vi "RefreshXYGraphV2.vi"(8 "error in (no error)":errorcluster caption="entrée d'erreur (pas d'erreur)", 9 "Graph Index":i32, 11 "Interface en entrée":refnum<class "Interface.lvclass"> caption="DNL_LabVIEW Object in") -> (0 "error out":errorcluster caption="sortie d'erreur", 1 "CurvesInd":i32[](array[numeric]), 2 "XYGraph_Ref":refnum<vi>, 3 "Interface en sortie":refnum<class "Interface.lvclass"> caption="DNL_LabVIEW Object out")   [LabVIEW 2010, in "Interface.lvclass"]
uses:
  Interface.lvclass
  Interface.lvclass/Interface.ctl
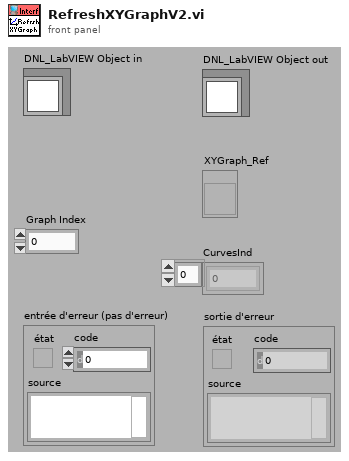
[diagram p1: front panel]
types:
  T1 = typedef "Interface.lvclass/CurveSetup.ctl" = cluster{"CurveName":string, "YParam":string, "XParam":string, "ZParam ":string, "GroupName":string, "LinWdth":u8, "PntCol":u32, "LinCol":u32, "LablFor":u8, "XScale":u32, "YScale":u32, "Interpol":u8, "DisplayName":string, "FillType":i16, "LineStyle":u8, "PntStyle":u8, "BarTyp":u8, "GraphIndex":i32, "Visible":bool, "XScaleName":string, "YScaleName":string, "XYGraph_Ref":refnum<vi>, "Data Only":bool, "DataQ Ref":refnum<queue>, "XParQ Ref":refnum<queue>}
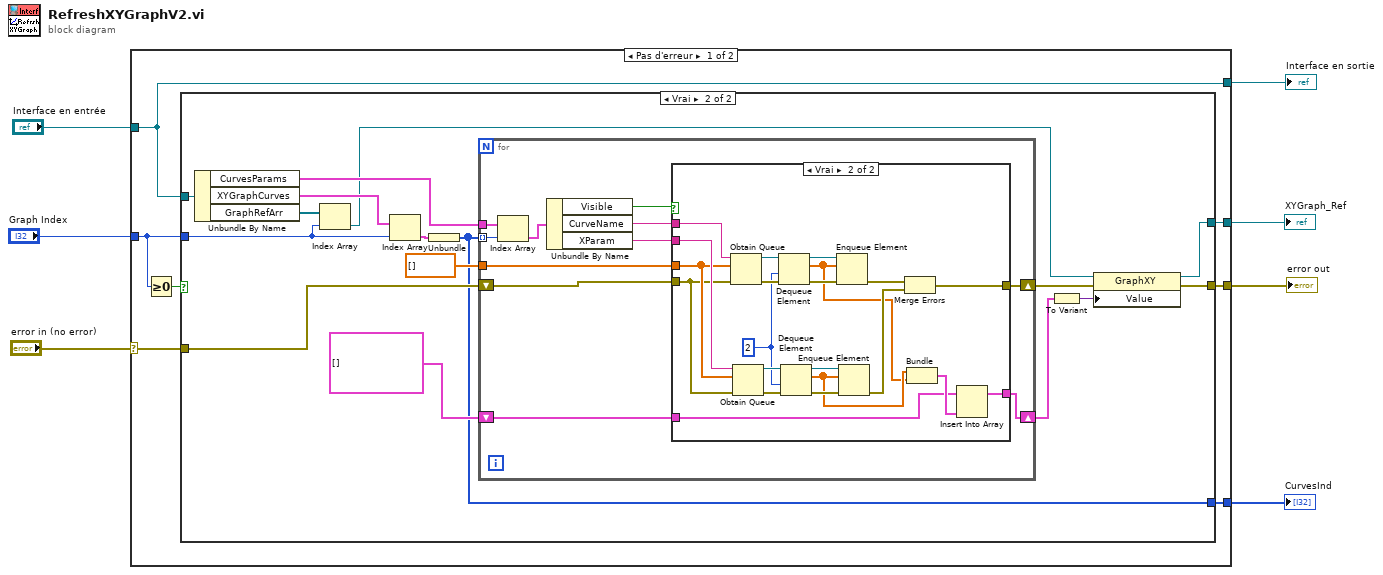
[diagram p0: block diagram]
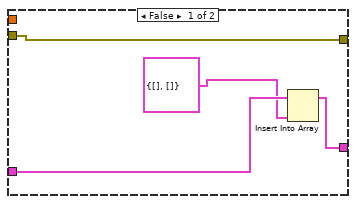
[diagram p3: hidden frame]
diagram:
  n1 = case shown="Pas d'erreur" "error in (no error)" {
    selector: "error in (no error)" -> [w13 w69]
    tunnel: [w12 w69] -> w6
    tunnel: [w14 w68] -> w4
    tunnel: "Interface en entrée" -> [w14 w68]
    tunnel: [w11 _] -> w3
    tunnel: [w10 _] -> w2
    tunnel: "Graph Index" -> [w9 _]
    frame No Error {
      n2 = Greater Or Equal To 0?(x=w9) -> (x >= 0?=w8:bool)
      n3 = case shown="Vrai" w8 {
        tunnel: w14 -> [_ w31]
        tunnel: w13 -> [w15 w29]
        tunnel: [w15 w20] -> w12
        tunnel: [_ w19] -> w11
        tunnel: [_ w26] -> w10
        tunnel: w9 -> [_ w25]
        frame False {
        }
        frame True {
          n4 = Unbundle By Name(w31) -> ("CurvesParams"=w22:T1[], "XYGraphCurves"=w23:cluster{"Tableau":i32[]}[], "GraphRefArr"=w24:refnum<vi>[])
          n5 = Index Array(array=w24, index=w25) -> (element=w17:refnum<vi>)
          n6 = Index Array(array=w23, index=w25) -> (element=w28:cluster{"Tableau":i32[]})
          n7 = Unbundle(w28) -> ("Tableau"=w26:i32[])
          n8 = for {
            tunnel: dbl[] [] -> [w38]
            tunnel: w26 -> [w41] mode=indexing
            shift-right: [w36] -> w18
            shift-left: w29 -> [w37]
            tunnel: w22 -> [w42]
            shift-right: [w34] -> w21
            shift-left: cluster{dbl[], dbl[]}[] [] -> [w35]
            n9 = Index Array(array=w42, index=w41) -> (element=w40:T1)
            n10 = Unbundle By Name(w40) -> ("Visible"=w32:bool, "CurveName"=w33:string, "XParam"=w39:string)
            n11 = case shown="Vrai" w32 {
              tunnel: w33 -> [_ w62]
              tunnel: w39 -> [_ w57]
              tunnel: w38 -> [_ w54]
              tunnel: w37 -> [w46 w53]
              tunnel: [w45 w52] -> w34
              tunnel: [w46 w56] -> w36
              tunnel: w35 -> [w44 w50]
              frame False {
                n12 = Insert Into Array(array=w44, new element=cluster{dbl[], dbl[]} {[], []} ("nouvel élément/sous-tableau")) -> (w45:cluster{dbl[], dbl[]}[])  [unwired: 1 in]
              }
              frame True {
                w47 = 2 ("timeout en ms (-1)")
                n13 = Obtain Queue(name (unnamed)=w62, element data type=w54, error in (no error)=w53) -> (queue out=w64:refnum<queue>, error out=w65:errorcluster)  [unwired: 2 in, 1 out]
                n14 = Obtain Queue(name (unnamed)=w57, element data type=w54, error in (no error)=w53) -> (queue out=w61:refnum<queue>, error out=w60:errorcluster)  [unwired: 2 in, 1 out]
                n15 = Dequeue Element(queue=w64, timeout in ms (-1)=w47, error in (no error)=w65) -> (queue out=w67:refnum<queue>, element=w48:dbl[], error out=w66:errorcluster)  [unwired: 1 out]
                n16 = Dequeue Element(queue=w61, timeout in ms (-1)=w47, error in (no error)=w60) -> (queue out=w58:refnum<queue>, element=w49:dbl[], error out=w59:errorcluster)  [unwired: 1 out]
                n17 = Enqueue Element(queue=w67, element=w48, error in (no error)=w66) -> (error out=w63:errorcluster)  [unwired: 1 in, 2 out]
                n18 = Enqueue Element(queue=w58, element=w49, error in (no error)=w59) -> (error out=w55:errorcluster)  [unwired: 1 in, 2 out]
                n19 = Merge Errors(w63, w55) -> (w56:errorcluster)
                n20 = Bundle(w49, w48) -> (w51:cluster{dbl[], dbl[]})  [unwired: 1 in]
                n21 = Insert Into Array(array=w50, new element=w51) -> (w52:cluster{dbl[], dbl[]}[])  [unwired: 1 in]
              }
            }
          }
          n22 = To Variant(anything=w21) -> (Variant=w16:variant)
          n23 = property on="Nœud de propriété" class="GraphXY"(reference=w17, error in=w18, "Value"=w16) -> (reference out=w19:refnum<vi>, error out=w20:errorcluster)
        }
      }
    }
    frame Error {
    }
  }
  "error out" <- w6
  "Interface en sortie" <- w4
  "XYGraph_Ref" <- w3
  "CurvesInd" <- w2
